vi "Update XY Graph.vi"(8 "error in (no error)":errorcluster, 10 "Current Position Y":dbl, 11 "Current Position X":dbl) -> (0 "error out":errorcluster, 2 "Array":T1(array[cluster]), 3 "String":string)   [LabVIEW 2022 SP3]
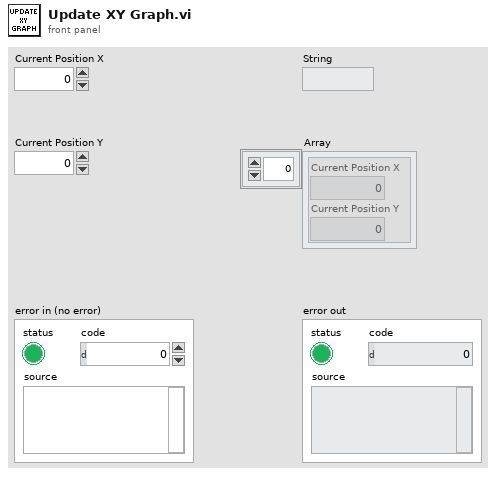
[diagram p1: front panel]
types:
  T1 = cluster{"Current Position X":dbl, "Current Position Y":dbl}[]
  T2 = cluster{"Current Position X":dbl, "Current Position Y":dbl}
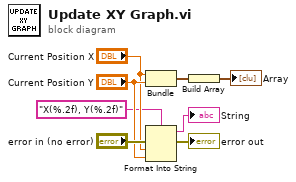
[diagram p0: block diagram]
diagram:
  n1 = Bundle("Current Position X"="Current Position X", "Current Position Y"="Current Position Y") -> (w1:T2)  [unwired: 1 in]
  n2 = Format Into String(format string="X(%.2f), Y(%.2f)", error in="error in (no error)", "Current Position X", "Current Position Y") -> (resulting string=→"String":string, error out=→"error out":errorcluster)  [unwired: 1 in]
  n3 = Build Array(w1) -> (→"Array":T1)
